vi "Map_ReadValue.vi"(10 "Address":u32, 11 "Plane":u8) -> (3 "Value":u8)   [LabVIEW 2020]
uses:
  <vilib>/Utility/file.llb/Application Directory.vi
  <vilib>/rvi/DataTransferAndStorage/Container/XNode/niFpgaContainer.xnode
  <vilib>/rvi/Memory/Memory_Emulation/nirvimemoryFastEmulation.vi
  <vilib>/rvi/Memory/Memory_Emulation/nirvimemoryEmulation.vi
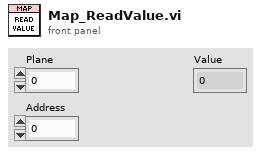
[diagram p1: front panel]
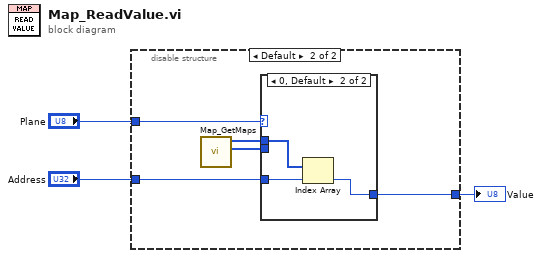
[diagram p0: block diagram]
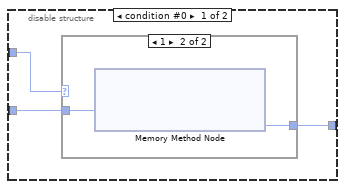
[diagram p2: hidden frame]
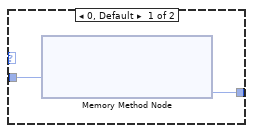
[diagram p3: hidden frame]
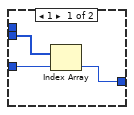
[diagram p4: hidden frame]
diagram:
  n1 = disable-structure shown="Default" {
    disable-tunnel: "Address" -> [w6 w15]
    disable-tunnel: [w5 w14] -> w3
    disable-tunnel: "Plane" -> [w4 w13]
    frame condition #0 {
      n2 = case shown="1" w4 {
        tunnel: w6 -> [w8 w10]
        tunnel: [w7 w9] -> w5
        frame 0, Default {
          n3 = xnode ("Memory Method Node")("Address"=w8) -> ("Data"=w7:u8)  [unwired: 1 in, 1 out]
        }
        frame 1 {
          n4 = xnode ("Memory Method Node")("Address"=w10) -> ("Data"=w9:u8)  [unwired: 1 in, 1 out]
        }
      }
    }
    frame condition #1 (active) {
      n5 = call "Map_GetMaps.vi"() -> ("Map Plane 1"=w12:u8[], "Map Plane 0"=w11:u8[])  [unwired: 10 in]
      n6 = case shown="0, Default" w13 {
        tunnel: w15 -> [w18 w21]
        tunnel: [w17 w20] -> w14
        tunnel: w12 -> [w16 _]
        tunnel: w11 -> [_ w19]
        frame 1 {
          n7 = Index Array(array=w16, index=w18) -> (element=w17:u8)
        }
        frame 0, Default {
          n8 = Index Array(array=w19, index=w21) -> (element=w20:u8)
        }
      }
    }
  }
  "Value" <- w3
